vi "Generate Firmware Libraries.vi"() -> ()   [LabVIEW 2014, in "LMH-LINX.lvlib"]
uses:
  vi.lib/MakerHub/LINX/LMH-LINX.lvlib
  <vilib>/MakerHub/Toolbox/LMH-Toolbox.lvlib
panel:
  out "Error Out":errorcluster
  in  "Libraries Destination Directory":path=path "C:/Users/samkristoff/Documents/Arduino/libraries"
  in  "Cancel Button":bool
  in  "Generate Button":bool
  # "This wizard will copy the LINX firmware source libraries into the directory you specify.\n\nNote: This is only necissary if you want to buid the LINX firmware from source code.\n\nDefault libraries locations:\nArduino IDE      C:\\Users\\<username>\\Documents\\Arduino\\libraries\nMPIDE                C:\\Users\\<username>\\Documents\\mpide\\libraries"
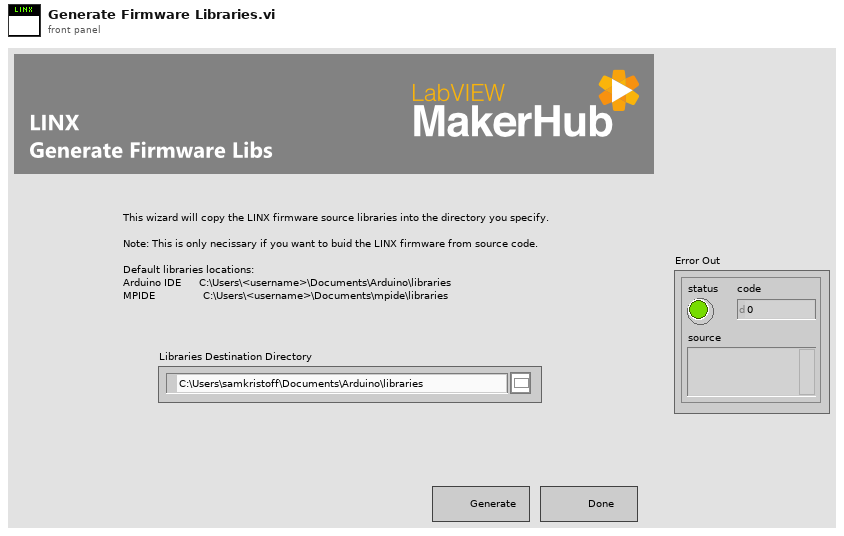
[diagram p1: front panel]
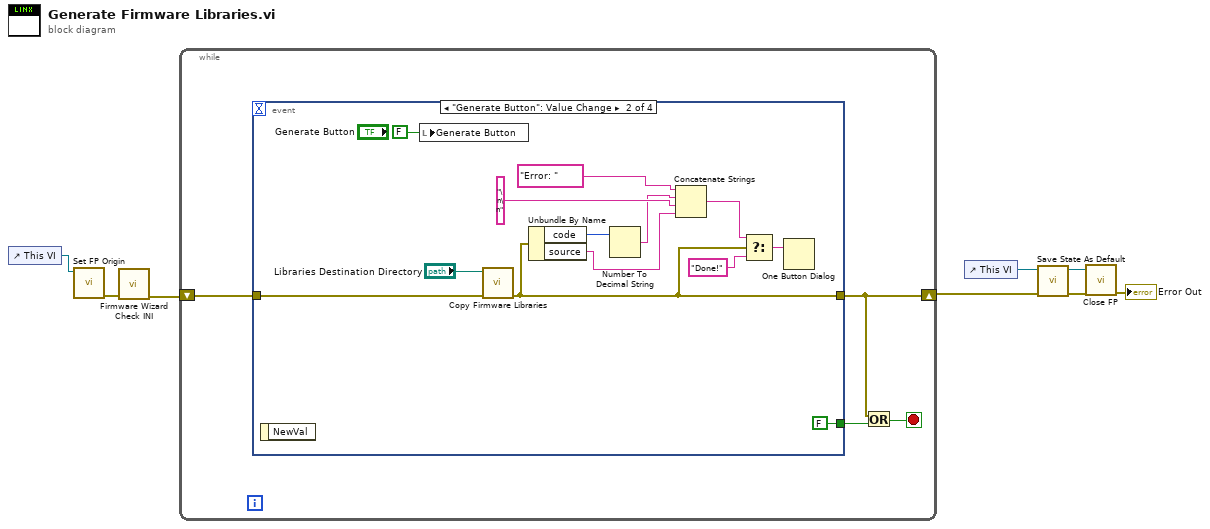
[diagram p0: block diagram]
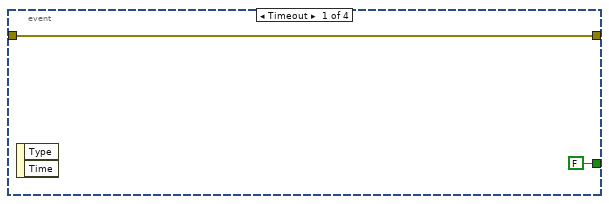
[diagram p2: hidden frame]
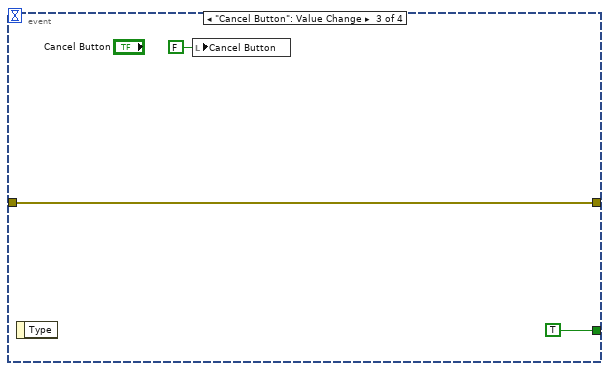
[diagram p3: hidden frame]
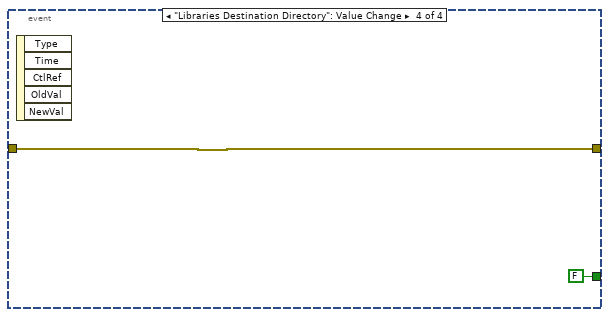
[diagram p4: hidden frame]
diagram:
  n1 = control-ref of="This VI"() -> (w8:refnum<vi>)
  n2 = call <vilib>:"Set FP Origin.vi"("VI Ref"=w8) -> ("Error Out"=w2:errorcluster)  [unwired: 10 in]
  n3 = call "Firmware Wizard Check INI.vi"("Error In"=w2) -> ("Error Out"=w1:errorcluster)  [unwired: 10 in]
  n4 = while {
    shift-right: [w9] -> w7
    shift-left: w1 -> [w12]
    stop <- w10 stop-if-true
    n5 = event shown="[1] \"Generate Button\": Value Change" {
      selector: _ -> [_ _ _ _]
      dyn-events: _ -> [_ _ _ _]
      timeout: _ -> [_ _ _ _]
      tunnel: w12 -> [w14 w26 w28 w31]
      tunnel: [FALSE ("Cancel Button") FALSE ("Cancel Button") TRUE ("Cancel Button") FALSE ("Cancel Button")] -> w11
      tunnel: [w14 w19 w28 w31] -> w9
      event Timeout {
        n6 = event-data() -> ()  [unwired: 1 in, 2 out]
      }
      event "Generate Button": Value Change {
        n7 = event-data() -> ()  [unwired: 1 in, 1 out]
        n8 = local write "Generate Button"(FALSE ("Generate Button")) -> ()
        n9 = call "Copy Firmware Libraries.vi"("Error In"=w26, "Library Destination Dir"="Libraries Destination Directory") -> ("Error Out"=w19:errorcluster)  [unwired: 9 in]
        n10 = Unbundle By Name(w19) -> ("code"=w23:i32, "source"=w18:string)
        n11 = Number To Decimal String(number=w23) -> (decimal integer string=w15:string)  [unwired: 1 in]
        n12 = Concatenate Strings("Error: " ("message"), w15, "\n\n" ("string"), w18) -> (w22:string)
        n13 = Select(t=w22, s=w19, f="Done!" ("message")) -> (s? t:f=w20:string)
        n14 = One Button Dialog(message=w20) -> ()  [unwired: 1 in, 1 out]
      }
      event "Cancel Button": Value Change {
        n15 = event-data() -> ()  [unwired: 1 in, 1 out]
        n16 = local write "Cancel Button"(FALSE ("Cancel Button")) -> ()
      }
      event "Libraries Destination Directory": Value Change {
        n17 = event-data() -> ()  [unwired: 1 in, 5 out]
      }
    }
    n18 = Or(x=w9, y=w11) -> (x .or. y?=w10:bool)
  }
  n19 = control-ref of="This VI"() -> (w6:refnum<vi>)
  n20 = call <vilib>:"Save State As Default.vi"("Error In"=w7, "Target VI"=w6) -> ("Error Out"=w4:errorcluster, "Target VI"=w5:refnum<vi>)  [unwired: 8 in]
  n21 = call <vilib>:"Close FP.vi"("Error In"=w4, "VI Ref"=w5) -> ("Error Out"=→"Error Out":errorcluster)  [unwired: 9 in]
